vi "hz to msec.vi"(11 "Loop Rate Hz":dbl) -> (3 "msec":u32)   [LabVIEW 2020]
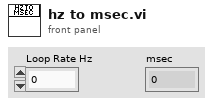
[diagram p1: front panel]
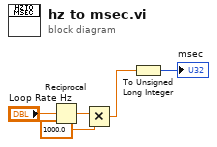
[diagram p0: block diagram]
diagram:
  n1 = Reciprocal(x="Loop Rate Hz") -> (1/x=w2:dbl)
  n2 = Multiply(x=w2, y=1000.0) -> (x*y=w4:dbl)
  n3 = To Unsigned Long Integer(number=w4) -> (unsigned 32bit integer=→"msec":u32)
